vi "writeToXML.vi"(8 "error in (no error)":errorcluster, 10 "ClassLabel":string, 11 "ProperMotion in":refnum<class "ProperMotion.lvclass">) -> (0 "error out":errorcluster, 2 "XMLout":string, 3 "ProperMotion out":refnum<class "ProperMotion.lvclass">)   [LabVIEW 2022 SP3, in "TCSDataDefinitions.lvlib" / "TCSCommand.lvlib" / "TargetConfiguration.lvlib" / "Target.lvlib" / "FixedTarget.lvlib" / "ProperMotion.lvclass"]
uses:
  ProperMotion.lvclass
  <userlib>/Common/UnitsAndXML/FlattenItemWithUnitToXML/FlattenAngularVelocityToXML/AngularVelocityUnit.ctl
  ProperMotion.lvclass/ProperMotion.ctl
  <userlib>/Common/UnitsAndXML/UnitsAndXML.lvlib
  <userlib>/Common/XML/XMLGenerator/XMLGenerator.lvclass
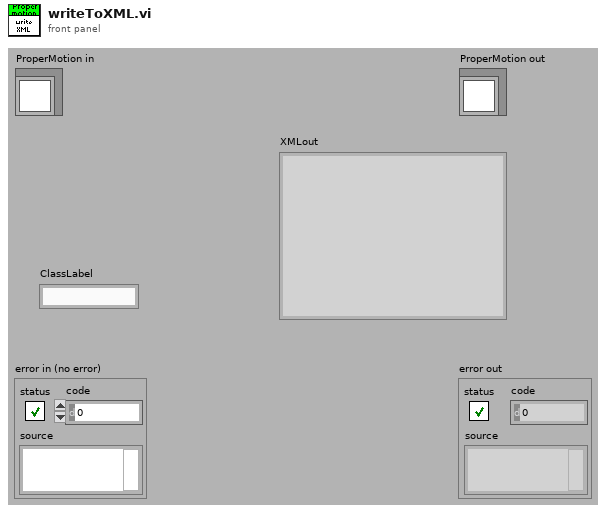
[diagram p1: front panel]
types:
  T1 = typedef "UnitsAndXML.lvlib/AngularVelocityUnit.ctl" = enum16{"\"/a", "deg/s", "\"/s"}
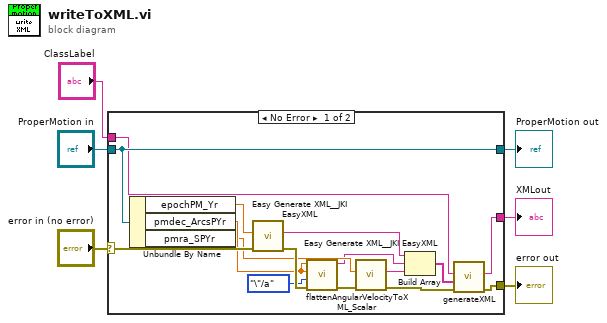
[diagram p0: block diagram]
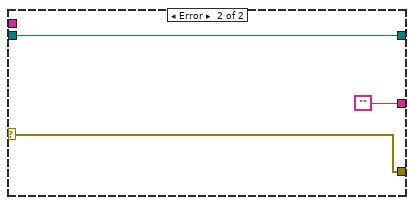
[diagram p2: hidden frame]
diagram:
  n1 = case shown="No Error" "error in (no error)" {
    selector: "error in (no error)" -> [w20 w25]
    tunnel: [w8 w25] -> w5
    tunnel: [w22 w24] -> w3
    tunnel: "ProperMotion in" -> [w22 w24]
    tunnel: "ClassLabel" -> [w10 _]
    tunnel: [w7 ""] -> w1
    frame No Error {
      n2 = Unbundle By Name(w22) -> ("epochPM_Yr"=w21:dbl, "pmdec_ArcsPYr"=w17:dbl[unit], "pmra_SPYr"=w15:dbl[unit])
      n3 = call <vilib>:"Easy Generate XML__JKI EasyXML.vi"("error in (no error)"=w20, "LabVIEW Data"=w21) -> ("error out"=w19:errorcluster, "XML String"=w12:string)  [unwired: 8 in]
      n4 = call <userlib>:"flattenAngularVelocityToXML_Scalar.vi"("error in (no error)"=w19, "angularVelocityUnitInXML"=AngularVelocityUnit."\"/a", "anuglarVelocityAgain"=w17, "angularVelocity"=w17) -> ("error out"=w18:errorcluster, "xmlString"=w13:string)  [unwired: 6 in]
      n5 = call <vilib>:"Easy Generate XML__JKI EasyXML.vi"("error in (no error)"=w18, "LabVIEW Data"=w15) -> ("error out"=w9:errorcluster, "XML String"=w14:string)  [unwired: 8 in]
      n6 = Build Array(w12, w13, w14) -> (w11:string[])
      n7 = call <userlib>:"generateXML.vi"("error in"=w9, "childrenXML"=w11, "elementName"=w10) -> ("error out"=w8:errorcluster, "XML out"=w7:string)  [unwired: 6 in, 1 out]
    }
    frame Error {
    }
  }
  "error out" <- w5
  "ProperMotion out" <- w3
  "XMLout" <- w1
